vi "search boolean array.vi"(2 "Previous Array":bool[](array[boolean]), 3 "Array In":bool[](array[boolean])) -> (0 "Array Out":bool[](array[boolean]), 1 "Index":i32)   [LabVIEW 2014]
panel:
  # "Find the Newest True Value in a Boolean Array"
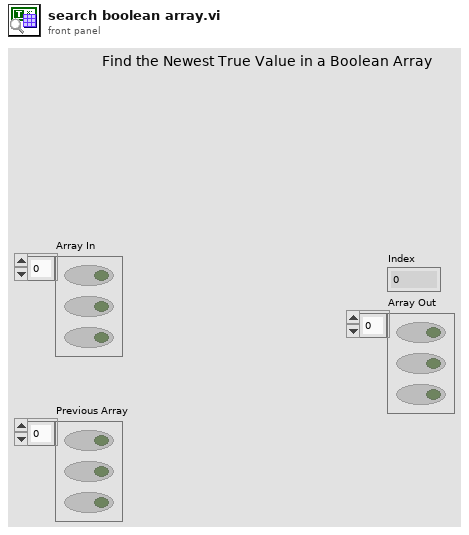
[diagram p1: front panel]
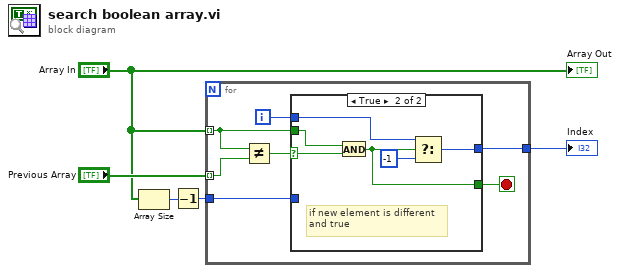
[diagram p0: block diagram]
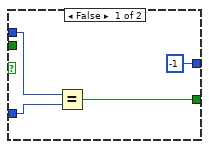
[diagram p2: hidden frame]
diagram:
  n1 = Array Size(array="Array In") -> (size(s)=w2:i32)
  n2 = Decrement(x=w2) -> (x-1=w1:i32)
  n3 = for {
    tunnel: "Array In" -> [w9] mode=indexing
    tunnel: "Previous Array" -> [w12] mode=indexing
    tunnel: [w10] -> w4
    tunnel: w1 -> [w6]
    i -> [w8]
    stop <- w7 stop-if-true
    n4 = Not Equal?(x=w9, y=w12) -> (x != y?=w11:bool)
    n5 = case shown="True" w11 {
      selector: w11 -> [_ w22]
      tunnel: [-1 ("f") w18] -> w10
      tunnel: w9 -> [_ w21]
      tunnel: w8 -> [w15 w20]
      tunnel: [w13 w17] -> w7
      tunnel: w6 -> [w14 _]
      frame False {
        n6 = Equal?(x=w15, y=w14) -> (x = y?=w13:bool)
      }
      frame True {
        # "if new element is different\nand true"
        n7 = And(x=w21, y=w22) -> (x .and. y?=w17:bool)
        n8 = Select(t=w20, s=w17, f=-1) -> (s? t:f=w18:i32)
      }
    }
  }
  "Index" <- w4
  "Array Out" <- "Array In"
